vi "InitBeforePage.vi"(4 "Header Footer Table Konfig":T5={"Header"={"Table Settings"={"Number of Columns"=2, "Width (%)"=100.0, "Relative Column Widths (%)"=[80.0, 20.0], "Horizontal Align"=0, "Header Rows"=0}, "Cell Defaults"={"Background Color"=16777215, "Horizontal Align"=3, "Vertical Align"=1, "Minimum Height"=0.0, "Fixed Height"=0.0, "Padding"={"Left"=2.0, "Top"=2.0, "Right"=2.0, "Bottom"=3.0}}, "Borders"={"Left"={"Enabled"=FALSE, "Width"=1.0, "Color"=0}, "Top"={"Enabled"=FALSE, "Width"=1.0, "Color"=0}, "Right"={"Enabled"=FALSE, "Width"=1.0, "Color"=0}, "Bottom"={"Enabled"=FALSE, "Width"=1.0, "Color"=0}, "Middle Horizontal"={"Enabled"=FALSE, "Width"=0.5, "Color"=0}, "Middle Vertical"={"Enabled"=FALSE, "Width"=0.5, "Color"=0}}}, "Footer"={"Table Settings"={"Number of Columns"=3, "Width (%)"=100.0, "Relative Column Widths (%)"=[15.0, 70.0, 15.0], "Horizontal Align"=0, "Header Rows"=0}, "Cell Defaults"={"Background Color"=16777215, "Horizontal Align"=0, "Vertical Align"=1, "Minimum Height"=0.0, "Fixed Height"=0.0, "Padding"={"Left"=2.0, "Top"=2.0, "Right"=2.0, "Bottom"=3.0}}, "Borders"={"Left"={"Enabled"=FALSE, "Width"=1.0, "Color"=0}, "Top"={"Enabled"=FALSE, "Width"=1.0, "Color"=0}, "Right"={"Enabled"=FALSE, "Width"=1.0, "Color"=0}, "Bottom"={"Enabled"=FALSE, "Width"=1.0, "Color"=0}, "Middle Horizontal"={"Enabled"=FALSE, "Width"=0.5, "Color"=0}, "Middle Vertical"={"Enabled"=FALSE, "Width"=0.5, "Color"=0}}}, "Footer Logo Row"={"Table Settings"={"Number of Columns"=1, "Width (%)"=100.0, "Relative Column Widths (%)"=[100.0], "Horizontal Align"=0, "Header Rows"=0}, "Cell Defaults"={"Background Color"=16777215, "Horizontal Align"=0, "Vertical Align"=1, "Minimum Height"=0.0, "Fixed Height"=0.0, "Padding"={"Left"=2.0, "Top"=2.0, "Right"=2.0, "Bottom"=3.0}}, "Borders"={"Left"={"Enabled"=FALSE, "Width"=1.0, "Color"=0}, "Top"={"Enabled"=FALSE, "Width"=1.0, "Color"=0}, "Right"={"Enabled"=FALSE, "Width"=1.0, "Color"=0}, "Bottom"={"Enabled"=FALSE, "Width"=1.0, "Color"=0}, "Middle Horizontal"={"Enabled"=FALSE, "Width"=0.5, "Color"=0}, "Middle Vertical"={"Enabled"=FALSE, "Width"=0.5, "Color"=0}}}} {"Footer Logo Row"."Cell Defaults"."Vertical Align" items=["Bottom", "Middle", "Top"]; "Footer Logo Row"."Cell Defaults"."Horizontal Align" items=["Center", "Justified", "JustifiedAll", "Left", "Right"]; "Footer Logo Row"."Table Settings"."Horizontal Align" items=["Center"=0, "Left"=3, "Right"=4]; "Footer"."Cell Defaults"."Vertical Align" items=["Bottom", "Middle", "Top"]; "Footer"."Cell Defaults"."Horizontal Align" items=["Center", "Justified", "JustifiedAll", "Left", "Right"]; "Footer"."Table Settings"."Horizontal Align" items=["Center"=0, "Left"=3, "Right"=4]; "Header"."Cell Defaults"."Vertical Align" items=["Bottom", "Middle", "Top"]; "Header"."Cell Defaults"."Horizontal Align" items=["Center", "Justified", "JustifiedAll", "Left", "Right"]; "Header"."Table Settings"."Horizontal Align" items=["Center"=0, "Left"=3, "Right"=4]}, 5 "Header Footer OffsetCluster":T9={"Header Offset"=20.0, "Footer Offset"=120.0, "Margin"={"Left"=40.0, "Right"=40.0, "Top"=60.0, "Bottom"=160.0}}, 6 "Font":T6={"Font"="Arial", "Size"=10, "Colour"=0, "Bold"=FALSE, "Italic"=FALSE, "Underline"=FALSE, "Strikethrough"=FALSE, "Font Encoding"=enum."Cp1252, WinANSI"}, 7 "Info":T11={"Header Footer Text Cluster"={"Header Text"="Protokoll XYZ", "Footer Text"="IAG nG", "Time"="<TIMESTAMP yyyy-MM-dd>", "Page Number"="Page <P> of <PT>"}, "PDF Details"={"Title"="Test PDF", "Subject"="Versa Tabasco", "Keywords"="", "Author"="RIW", "Creator"="IAG"}}, 8 "Fehler (Eingang, kein Fehler)":errorcluster, 9 "Footer Image File Path":path, 10 "Header Image File Path":path, 11 "Path (Dialog if Empty)":path=path "D:/IAG_DATA/Log/Test Protokoll.pdf") -> (0 "Fehler (Ausgang)":errorcluster, 3 "Context (Ausgang)":refnum<class "Context.lvclass">)   [LabVIEW 2020, in "PDF Interface.lvlib"]
doc: "To create a PDF before adding content."
uses:
  PDF Interface.lvlib
  <vilib>/Simplicity AI/SAI_PDF_API/Classes/Context/Controls/SAI_PDF_PDF Details.ctl
  <vilib>/Simplicity AI/SAI_PDF_API/Classes/Context/Context.lvclass
  <vilib>/Simplicity AI/SAI_PDF_API/Classes/Context/Controls/SAI_PDF_Margins.ctl
  <vilib>/Simplicity AI/SAI_PDF_API/Classes/Context/Controls/SAI_PDF_Font.ctl
  <vilib>/Simplicity AI/SAI_PDF_API/Classes/Context/Controls/SAI_PDF_Font Encoding.ctl
  <vilib>/Simplicity AI/SAI_PDF_API/Classes/Table Builder/Controls/SAI_PDF_Table Configuration.ctl
  <vilib>/Simplicity AI/SAI_PDF_API/Classes/Table Builder/Controls/SAI_PDF_Table Horizontal Align.ctl
  <vilib>/Simplicity AI/SAI_PDF_API/Classes/Table Builder/Controls/SAI_PDF_Default Cell Format.ctl
  <vilib>/Simplicity AI/SAI_PDF_API/Classes/Table Builder/Controls/SAI_PDF_BorderLine.ctl
  PDF Interface Helper/PDF Interface Helper.lvlib
  <vilib>/Simplicity AI/SAI_PDF_API/Classes/Table Builder/Table Builder.lvclass
panel:
  # "(Cp1252)"
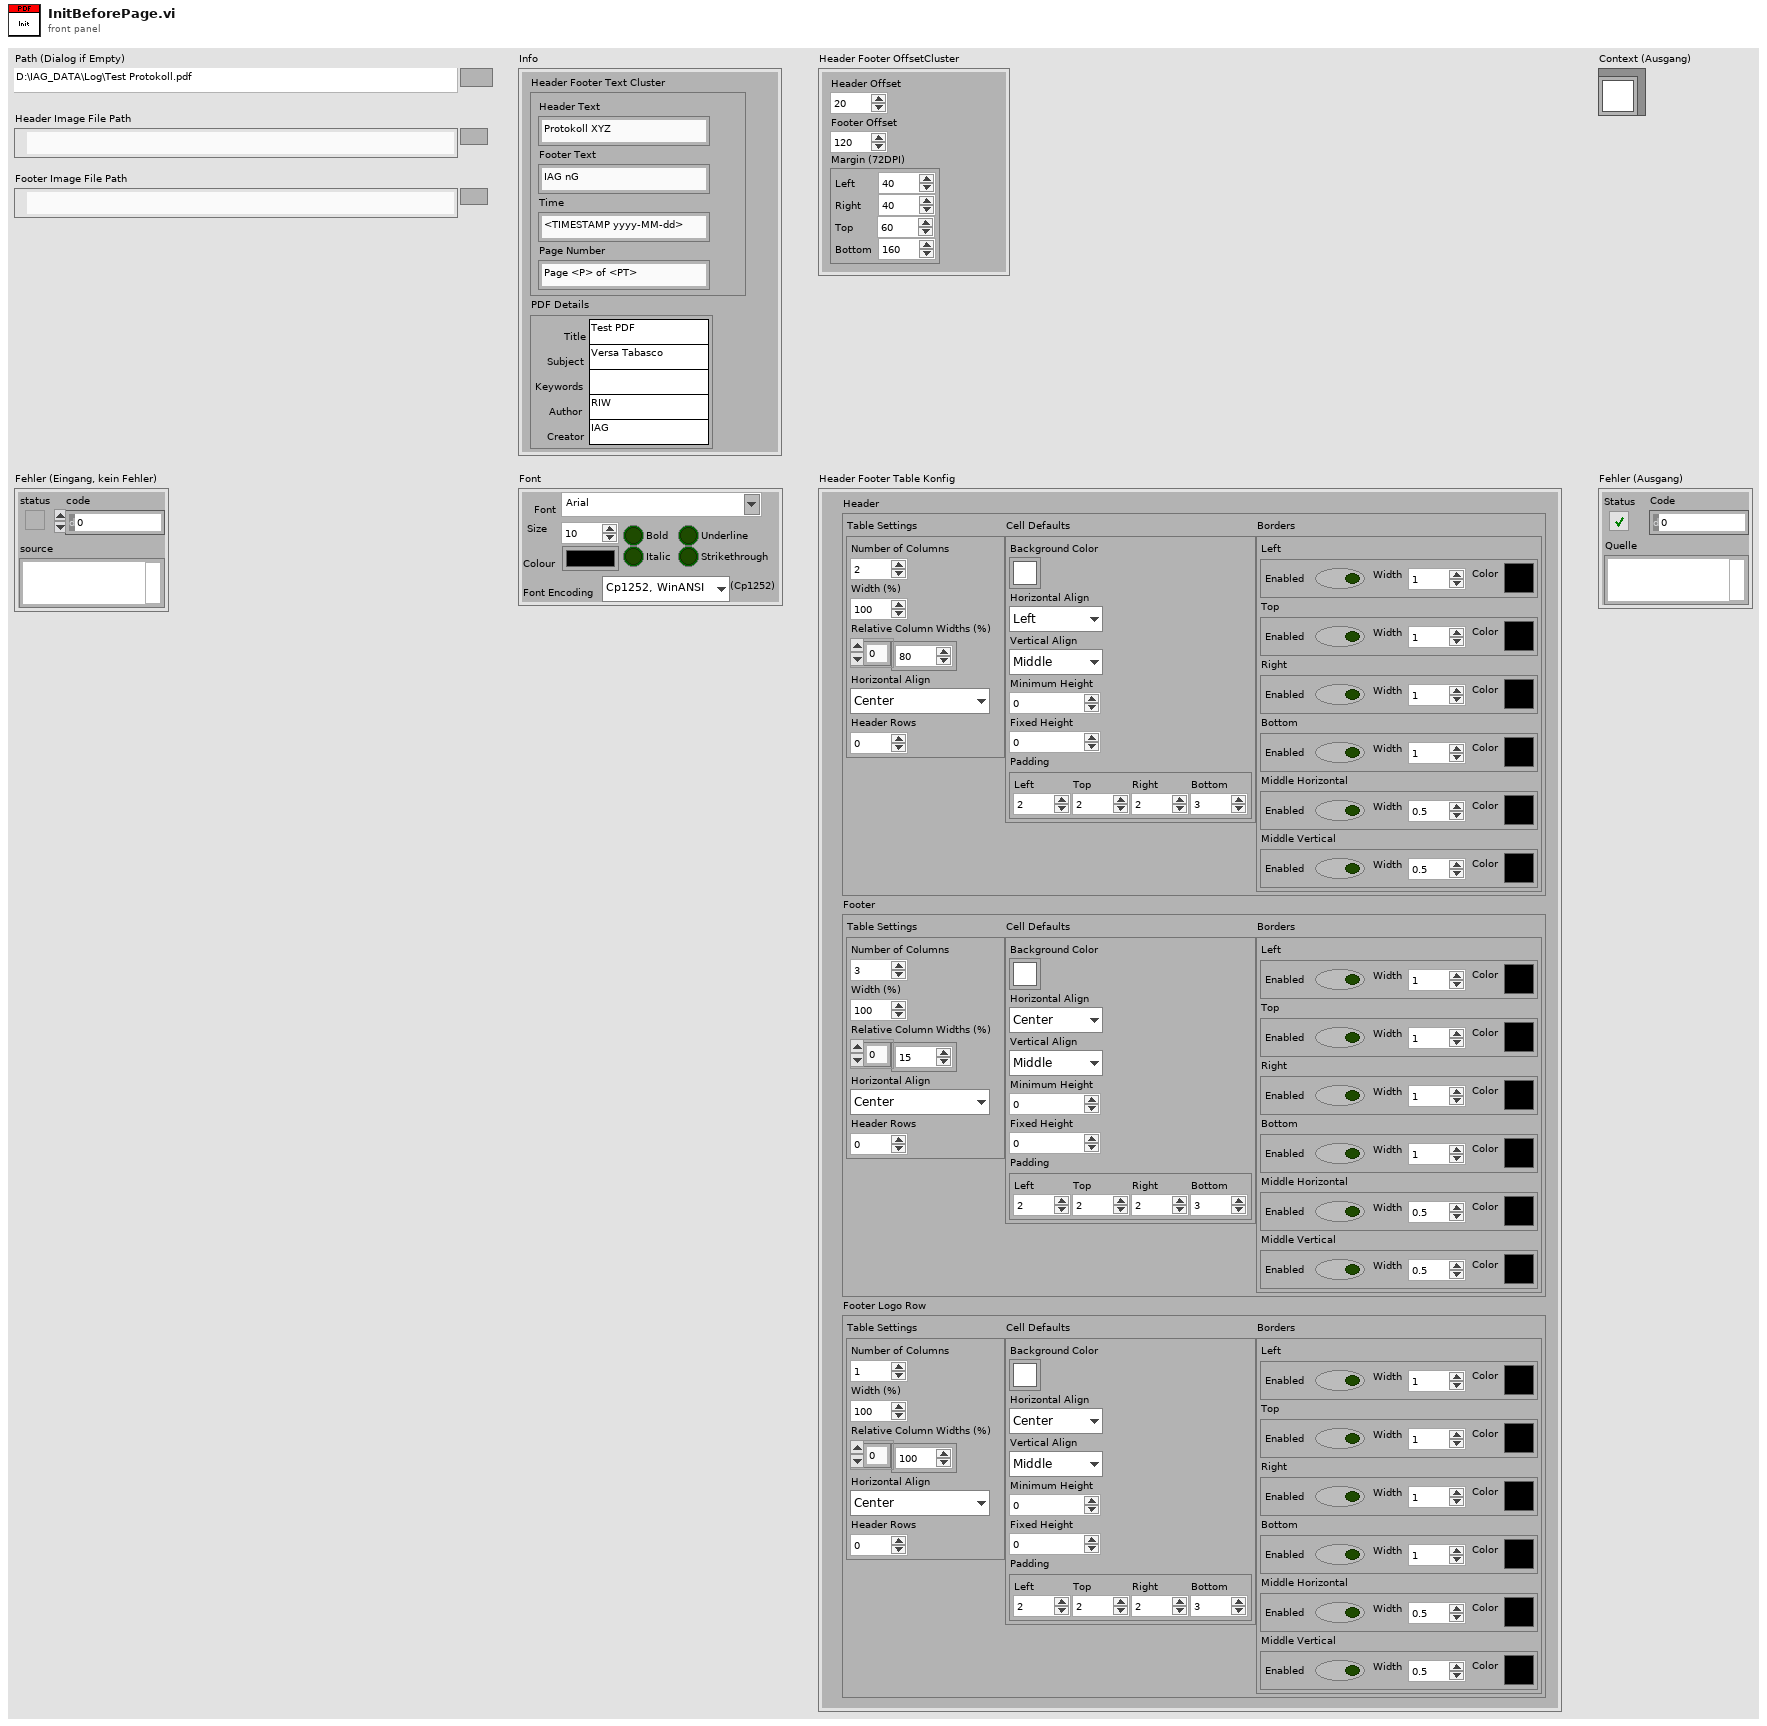
[diagram p1: front panel]
types:
  T1 = typedef "SAI_PDF_Toolkit.lvlib/Table Builder.lvclass/SAI_PDF_Table Configuration.ctl" = cluster{"Table Settings":cluster{"Number of Columns":i32, "Width (%)":sgl, "Relative Column Widths (%)":sgl[], "Horizontal Align":T2, "Header Rows":i32}, "Cell Defaults":T3, "Borders":cluster{"Left":T4, "Top":T4, "Right":T4, "Bottom":T4, "Middle Horizontal":T4, "Middle Vertical":T4}}
  T2 = typedef "SAI_PDF_Toolkit.lvlib/Table Builder.lvclass/SAI_PDF_Table Horizontal Align.ctl" = i32
  T3 = typedef "SAI_PDF_Toolkit.lvlib/Table Builder.lvclass/SAI_PDF_Default Cell Format.ctl" = cluster{"Background Color":u32, "Horizontal Align":i32, "Vertical Align":i32, "Minimum Height":sgl, "Fixed Height":sgl, "Padding":cluster{"Left":sgl, "Top":sgl, "Right":sgl, "Bottom":sgl}}
  T4 = typedef "SAI_PDF_Toolkit.lvlib/Table Builder.lvclass/SAI_PDF_BorderLine.ctl" = cluster{"Enabled":bool, "Width":sgl, "Color":u32}
  T5 = cluster{"Header":T1, "Footer":T1, "Footer Logo Row":T1}
  T6 = typedef "SAI_PDF_Toolkit.lvlib/Context.lvclass/SAI_PDF_Font.ctl" = cluster{"Font":string, "Size":i32, "Colour":u32, "Bold":bool, "Italic":bool, "Underline":bool, "Strikethrough":bool, "Font Encoding":T7}
  T7 = typedef "SAI_PDF_Toolkit.lvlib/Context.lvclass/SAI_PDF_Font Encoding.ctl" = enum16{"Cp1252, WinANSI", "IdentityH", "IdentityV", "Cp1250", "Cp1257", "MacRoman"}
  T8 = typedef "SAI_PDF_Toolkit.lvlib/Context.lvclass/SAI_PDF_Margins.ctl" = cluster{"Left":sgl, "Right":sgl, "Top":sgl, "Bottom":sgl}
  T9 = cluster{"Header Offset":sgl, "Footer Offset":sgl, "Margin":T8}
  T10 = typedef "SAI_PDF_Toolkit.lvlib/Context.lvclass/SAI_PDF_PDF Details.ctl" = cluster{"Title":string, "Subject":string, "Keywords":string, "Author":string, "Creator":string}
  T11 = cluster{"Header Footer Text Cluster":cluster{"Header Text":string, "Footer Text":string, "Time":string, "Page Number":string}, "PDF Details":T10}
  T12 = cluster{"Header Text":string, "Footer Text":string, "Time":string, "Page Number":string}
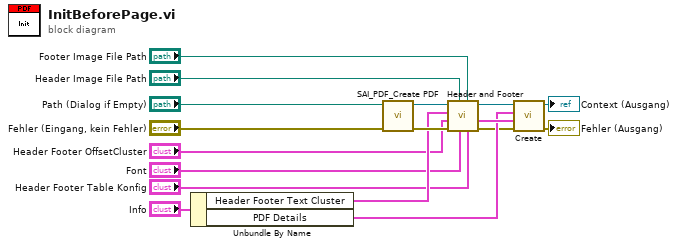
[diagram p0: block diagram]
diagram:
  n1 = Unbundle By Name("Info") -> ("Header Footer Text Cluster"=w4:T12, "PDF Details"=w16:T10)
  n2 = call <vilib>:"SAI_PDF_Create PDF.vi"("error in"="Fehler (Eingang, kein Fehler)", "Path (Dialog if Empty)"="Path (Dialog if Empty)") -> ("error out"=w6:errorcluster, "Context Out"=w7:refnum<class "Context.lvclass">)  [unwired: 2 in, 6 out]
  n3 = call "Header and Footer.vi"("Header Footer Table Konfig"="Header Footer Table Konfig", "Footer Image File Path"="Footer Image File Path", "Font"="Font", "Header Image File Path"="Header Image File Path", "error in"=w6, "Header Footer OffsetCluster"="Header Footer OffsetCluster", "Header Footer Text Cluster"=w4, "Context In"=w7) -> ("error out"=w8:errorcluster, "Header Footer OffsetCluster out"=w17:T9, "Context out"=w9:refnum<class "Context.lvclass">)  [unwired: 1 out]
  n4 = call "Create.vi"("error in"=w8, "Header Footer OffsetCluster"=w17, "PDF Details"=w16, "Context In"=w9) -> ("error out"=→"Fehler (Ausgang)":errorcluster, "Context Out"=→"Context (Ausgang)":refnum<class "Context.lvclass">)  [unwired: 6 out]
